vi "TCPIP.Server v2.vi"() -> ()   [LabVIEW 2014]
panel:
  in  "port":u16=50009
  in  "file (use dialog)":path=path "D:/DNN_data/20170731_testrun.txt"
  out "Client Connected":bool=TRUE
  out "Command (from Python)":string="hello(world)\r\n"
  out "Return Value String (for Python)":string="Hello world"
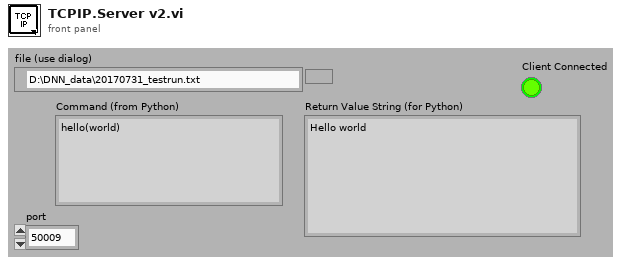
[diagram p1: front panel]
types:
  T1 = enum16{"Standard", "Buffered", "CRLF", "Immediate"}
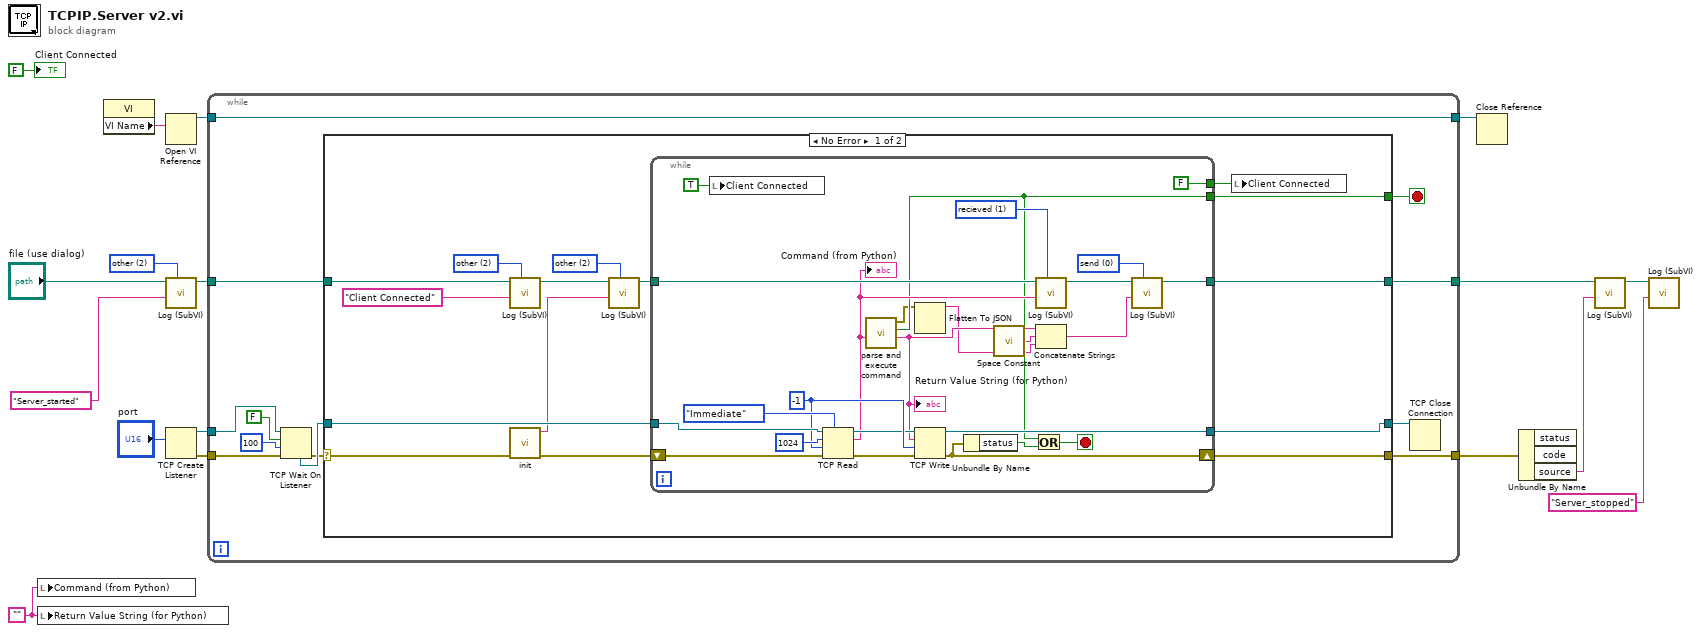
[diagram p0: block diagram]
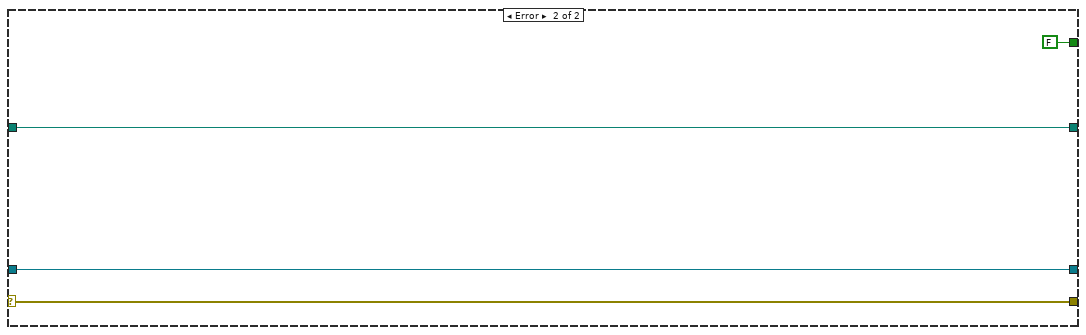
[diagram p2: hidden frame]
diagram:
  w7 = u16 2 items=["send", "recieved", "other"] ("Msgtype")
  w13 = ""
  n1 = local write "Command (from Python)"(w13) -> ()
  n2 = local write "Return Value String (for Python)"(w13) -> ()
  n3 = property class="VI"() -> ("VI Name"=w16:string)  [unwired: 2 in, 2 out]
  n4 = Open VI Reference(vi path=w16) -> (vi reference=w15:refnum<vi>)  [unwired: 5 in, 1 out]
  n5 = call "Log (SubVI).vi"("Msgtype"=w7, "String"="Server_started", "file path (use dialog)"="file (use dialog)") -> ("path"=w9:path)  [unwired: 8 in]
  n6 = TCP Create Listener(10:"port") -> (0:w17:errorcluster, 3:w10:refnum<k5>)  [unwired: 4 in, 1 out]
  n7 = while {
    tunnel: w15 -> [w24]
    tunnel: [w24] -> w14
    tunnel: w17 -> [w29]
    tunnel: w10 -> [w22]
    tunnel: w9 -> [w21]
    tunnel: [w20] -> w5
    tunnel: [w19] -> w4
    stop <- w18 stop-if-true
    n8 = TCP Wait On Listener(8:w29, 9:100 ("timeout ms (wait forever: -1)"), 10:FALSE ("resolve remote address (T)"), 11:w22) -> (0:w23:errorcluster, 4:w27:refnum<k5>)  [unwired: 3 out]
    n9 = case shown="No Error" w23 {
      selector: w23 -> [w38 w71]
      tunnel: w27 -> [w44 w73]
      tunnel: [w43 w73] -> w26
      tunnel: w21 -> [w33 w72]
      tunnel: [w41 w72] -> w20
      tunnel: [w40 w71] -> w19
      tunnel: [w39 FALSE ("exit")] -> w18
      frame No Error {
        w30 = u16 2 items=["send", "recieved", "other"] ("Msgtype")
        w35 = u16 2 items=["send", "recieved", "other"] ("Msgtype")
        n10 = call "Log (SubVI).vi"("Msgtype"=w30, "String"="Client Connected", "file path (use dialog)"=w33) -> ("path"=w32:path)  [unwired: 8 in]
        n11 = call "init.vi"("error in (no error)"=w38) -> ("error out"=w37:errorcluster, "Output"=w34:string)  [unwired: 9 in]
        n12 = call "Log (SubVI).vi"("Msgtype"=w35, "String"=w34, "file path (use dialog)"=w32) -> ("path"=w36:path)  [unwired: 8 in]
        n13 = while {
          tunnel: [FALSE ("Connected")] -> w42
          shift-left: w37 -> [w64]
          shift-right: [w63] -> w40
          tunnel: [w65] -> w43
          tunnel: w44 -> [w66]
          tunnel: w36 -> [w58]
          tunnel: [w54] -> w41
          tunnel: [w49] -> w39
          stop <- w50 stop-if-true
          w55 = u16 0 items=["send", "recieved", "other"] ("Msgtype")
          w56 = u16 1 items=["send", "recieved", "other"] ("Msgtype")
          w60 = -1 ("timeout ms (25000)")
          n14 = local write "Client Connected"(TRUE ("Connected")) -> ()
          n15 = TCP Read(connection ID=w66, bytes to read=1024, error in (no error)=w64, 7:T1."Immediate" ("mode (standard)"), 9:w60) -> (connection ID out=w59:refnum<k5>, data out=w53:string, error out=w67:errorcluster)
          "Command (from Python)" <- w53
          n16 = call "parse and execute command.vi"("Python Command"=w53) -> ("Python Return String"=w52:string, "exit"=w49:bool, "command error"=w46:errorcluster)  [unwired: 7 in]
          "Return Value String (for Python)" <- w52
          n17 = Flatten To JSON(anything=w46) -> (JSON string=w45:string)  [unwired: 2 in, 1 out]
          n18 = TCP Write(connection ID=w59, data in=w52, error in (no error)=w67, 9:w60) -> (connection ID out=w65:refnum<k5>, error out=w63:errorcluster)  [unwired: 1 out]
          n19 = Unbundle By Name(w63) -> ("status"=w51:bool)
          n20 = call <vilib>:"Space Constant.vi"() -> ("String"=w47:string)
          n21 = Or(x=w49, y=w51) -> (x .or. y?=w50:bool)
          n22 = call "Log (SubVI).vi"("Msgtype"=w56, "String"=w53, "file path (use dialog)"=w58) -> ("path"=w57:path)  [unwired: 8 in]
          n23 = Concatenate Strings(w52, w47, w45) -> (w48:string)
          n24 = call "Log (SubVI).vi"("Msgtype"=w55, "String"=w48, "file path (use dialog)"=w57) -> ("path"=w54:path)  [unwired: 8 in]
        }
        n25 = local write "Client Connected"(w42) -> ()
      }
      frame Error {
      }
    }
    n26 = TCP Close Connection(connection ID=w26) -> ()  [unwired: 2 in, 2 out]
  }
  n27 = Close Reference(reference=w14) -> ()  [unwired: 1 in, 1 out]
  n28 = Unbundle By Name(w4) -> ("source"=w3:string)  [unwired: 2 out]
  n29 = call "Log (SubVI).vi"("String"=w3, "file path (use dialog)"=w5) -> ("path"=w2:path)  [unwired: 9 in]
  n30 = call "Log (SubVI).vi"("String"="Server_stopped", "file path (use dialog)"=w2) -> ()  [unwired: 9 in, 1 out]
  "Client Connected" <- FALSE ("Connected")
